vi "WfrmBdcst.vi"(8 "error in (no error)":errorcluster, 10 "Waveforms":variant, 11 "Module":refnum<class "ModuleAdmin.lvclass">) -> (0 "error out":errorcluster, 3 "Module":refnum<class "ModuleAdmin.lvclass">)   [LabVIEW 2018, in "DigitizerPlugins.lvlib" / "DigitizerBase.lvclass"]
uses:
  DigitizerBase.lvclass
  <userlib>/NIST/ModuleAdminLib/ModuleAdmin/ModuleAdmin.lvclass
  DigitizerShared/clEventType.ctl
  DigitizerShared/DigitizerShared.lvlib
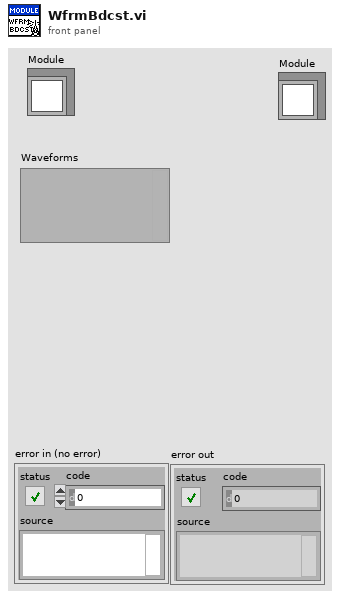
[diagram p1: front panel]
types:
  T1 = typedef "DigitizerShared.lvlib/clEventType.ctl" = cluster{"ModuleID":i32, "Data":variant}
  T2 = typedef "DigitizerShared.lvlib/clBroadcastEvents.ctl" = cluster{"DidInit":refnum<user-event>, "StatusUpdate":refnum<user-event>, "ErrorReport":refnum<user-event>, "DidStop":refnum<user-event>, "PathToINI":refnum<user-event>, "Channels":refnum<user-event>, "Acq":refnum<user-event>, "Trigger":refnum<user-event>, "Waveforms":refnum<user-event>}
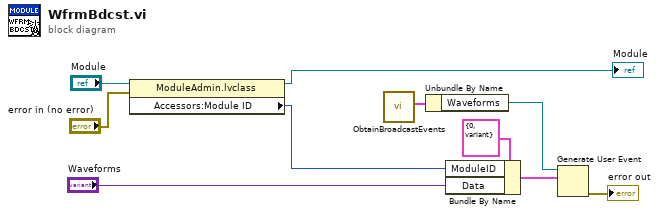
[diagram p0: block diagram]
diagram:
  n1 = property class="ModuleAdmin.lvclass"(reference="Module", error in="error in (no error)") -> (reference out=→"Module":refnum<class "ModuleAdmin.lvclass">, "Accessors:Module ID"=w4:i32)  [unwired: 1 out]
  n2 = call "ObtainBroadcastEvents.vi"() -> ("clDigitizerBdcstEvents"=w10:T2)  [unwired: 10 in, 1 out]
  n3 = Unbundle By Name(w10) -> ("Waveforms"=w9:refnum<user-event>)
  n4 = Bundle By Name(cluster=T1 {"ModuleID"=0, "Data"=variant} ("clBroadcast"), "ModuleID"=w4, "Data"="Waveforms") -> (w7:T1)
  n5 = Generate User Event(user event=w9, event data cluster=w7) -> (error out=→"error out":errorcluster)  [unwired: 2 in, 1 out]
